vi "log in.vi"(0 "路径":path, 5 "UserGroups in":enum16{"Operator", "Engineer", "Admin"}(ring), 11 "error in (no error)":errorcluster caption="错误输入（无错误）") -> (4 "State":T1, 6 "Giveup?":bool, 8 "UserGroups":enum16{"Operator", "Engineer", "Admin"}(ring), 10 "User":string, 15 "error out":errorcluster caption="错误输出")   [LabVIEW 2017]
uses:
  Regedit.ctl
panel:
  in  "Exit":bool
  in  "Account":bool
  in  "Regist":bool
  in  "Login":bool
  in  "登录":T2
  # "Login"
  # "Tips\n1. Register new users for the user group (the administrator account cannot be registered)\n2. Select the user group;\n3. Enter the user name and password\n4, login"
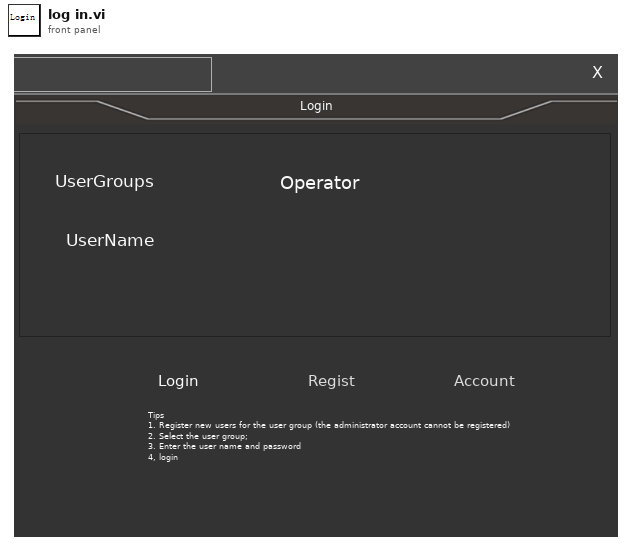
[diagram p1: front panel]
types:
  T1 = typedef "Regedit.ctl" = enum16{"Initialize", "Idle", "Judge", "Save", "Regedit", "Account", "Delete", "Sure?", "Stop"}
  T2 = cluster{"UserGroups":enum16{"Operator", "Engineer", "Admin"}, "UserName":string, "PassWord":string}
  T3 = enum8{"Enabled", "Disabled", "Disabled and Grayed Out"}
  T4 = enum16{"Operator", "Technician", "Engineer", "Developer"}
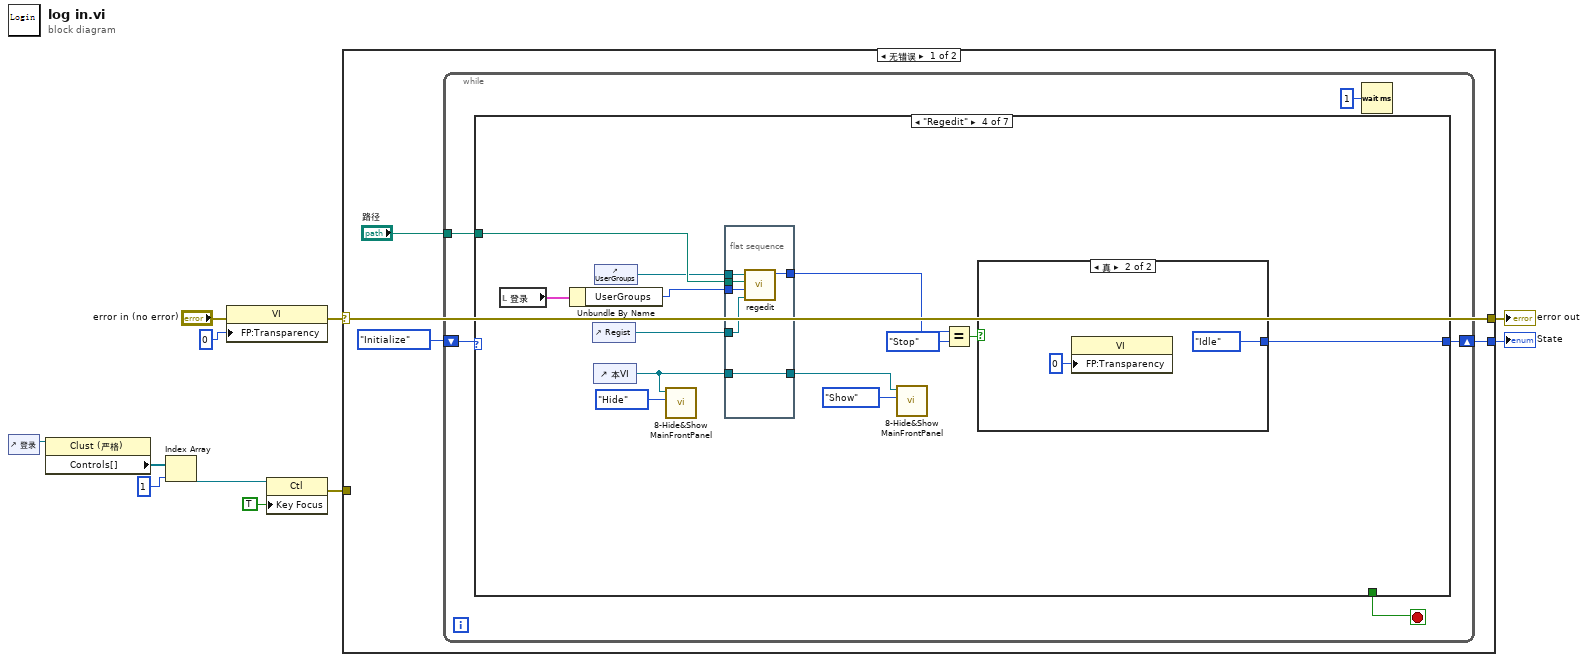
[diagram p0: block diagram]
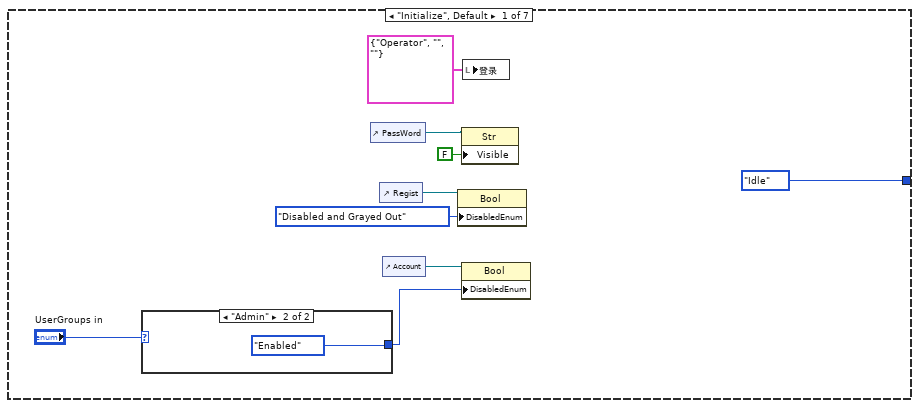
[diagram p2: hidden frame]
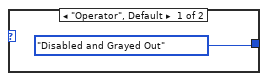
[diagram p3: hidden frame]
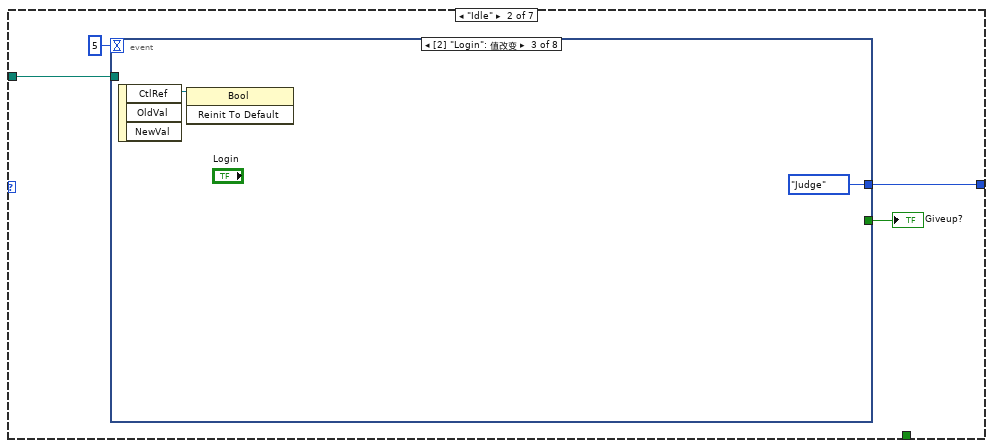
[diagram p4: hidden frame]
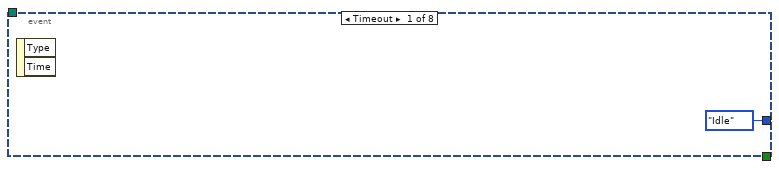
[diagram p5: hidden frame]
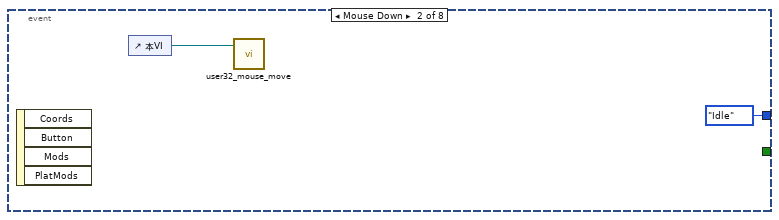
[diagram p6: hidden frame]
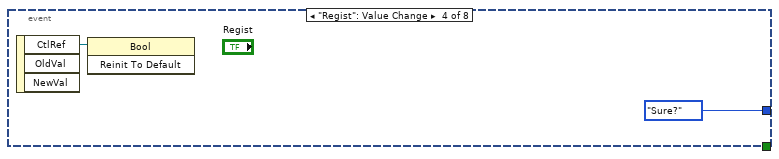
[diagram p7: hidden frame]
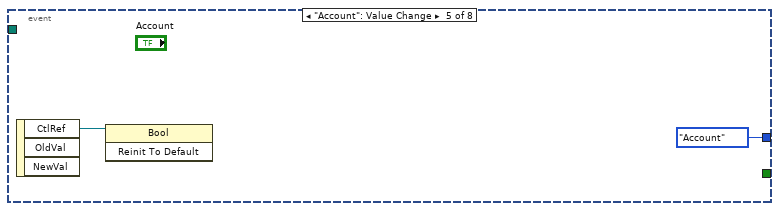
[diagram p8: hidden frame]
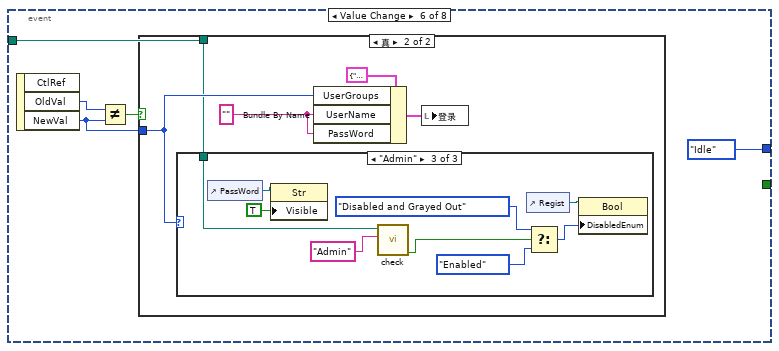
[diagram p9: hidden frame]
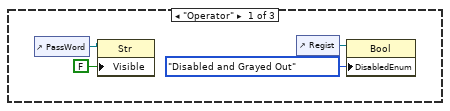
[diagram p11: hidden frame]
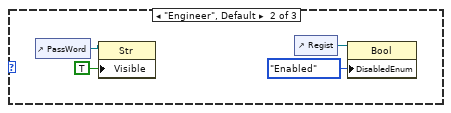
[diagram p12: hidden frame]
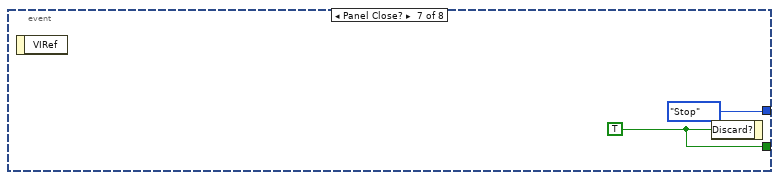
[diagram p13: hidden frame]
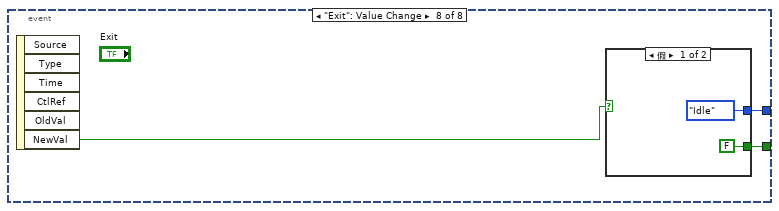
[diagram p14: hidden frame]
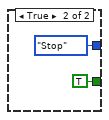
[diagram p15: hidden frame]
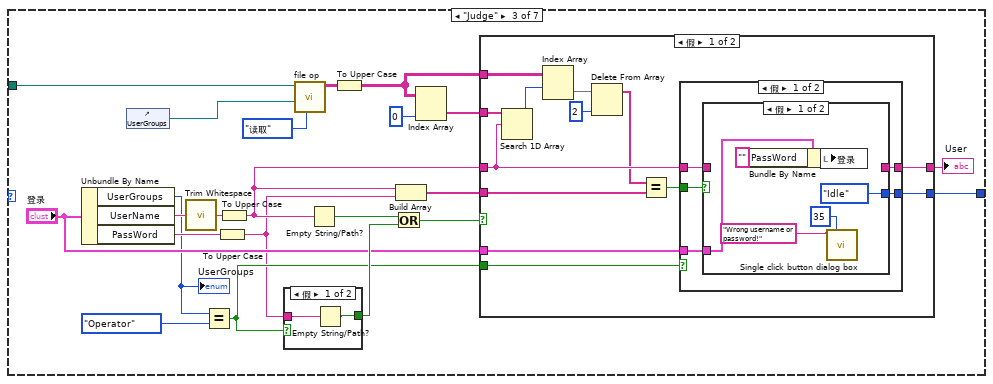
[diagram p16: hidden frame]
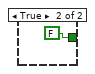
[diagram p17: hidden frame]
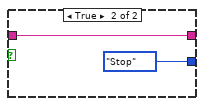
[diagram p18: hidden frame]
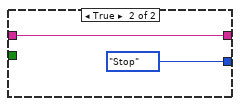
[diagram p19: hidden frame]
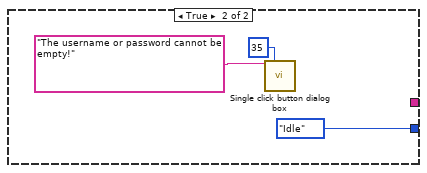
[diagram p20: hidden frame]
diagram:
  n1 = control-ref of="登录"() -> (w6:refnum<vi>)
  n2 = property class="Clust (严格)"(reference=w6) -> ("Controls[]"=w5:refnum<vi>[])  [unwired: 1 in, 2 out]
  n3 = Index Array(array=w5, index=1 ("索引")) -> (element=w3:refnum<vi>)
  n4 = property class="VI"(error in="error in (no error)", "FP:Transparency"=u8 0 ("前面板窗口:透明度")) -> (error out=w8:errorcluster)  [unwired: 1 in, 1 out]
  n5 = property class="Ctl"(reference=w3, "Key Focus"=TRUE ("键选中")) -> (error out=w1:errorcluster)  [unwired: 1 in, 1 out]
  n6 = case shown="无错误" w8 {
    selector: w8 -> [w14 w186]
    tunnel: [w14 w186] -> w11
    tunnel: [w13 _] -> w10
    tunnel: w1 -> [_ _]
    frame No Error {
      n7 = while {
        shift-right: [w19] -> w13
        shift-left: Regedit."Initialize" -> [w20]
        tunnel: "路径" -> [w17]
        stop <- w16 stop-if-true
        n8 = case shown="\"Regedit\"" w20 {
          tunnel: [Regedit."Idle" w34 w99 w146 Regedit."Idle" w168 Regedit."Stop"] -> w19
          tunnel: w17 -> [_ w32 w90 w145 w163 w169 _]
          tunnel: [_ _ _ _ _ _ TRUE] -> w16
          frame "Initialize", Default {
            n9 = case shown="\"Admin\"" "UserGroups in" {
              tunnel: [T3."Disabled and Grayed Out" ("禁用") T3."Enabled" ("禁用")] -> w22
              frame "Operator", Default {
              }
              frame "Admin" {
              }
            }
            n10 = control-ref of="PassWord"() -> (w28:refnum<vi>)
            n11 = control-ref of="Regist"() -> (w25:refnum<vi>)
            n12 = control-ref of="Account"() -> (w24:refnum<vi>)
            n13 = property class="Bool"(reference=w25, "DisabledEnum"=T3."Disabled and Grayed Out" ("禁用")) -> ()  [unwired: 1 in, 2 out]
            n14 = property class="Str"(reference=w28, "Visible"=FALSE ("可见")) -> ()  [unwired: 1 in, 2 out]
            n15 = property class="Bool"(reference=w24, "DisabledEnum"=w22) -> ()  [unwired: 1 in, 2 out]
            n16 = local write "登录"(T2 {"UserGroups"=enum."Operator", "UserName"="", "PassWord"=""} ("登录")) -> ()
          }
          frame "Idle" {
            n17 = event shown="[2] \"Login\": 值改变" {
              selector: _ -> [_ _ _ _ _ _ _ _]
              dyn-events: _ -> [_ _ _ _ _ _ _ _]
              timeout: 5 -> [_ _ _ _ _ _ _ _]
              tunnel: [Regedit."Idle" Regedit."Idle" Regedit."Judge" Regedit."Sure?" Regedit."Account" Regedit."Idle" Regedit."Stop" w76] -> w34
              tunnel: [_ _ _ _ _ _ w72 w75] -> w33
              tunnel: w32 -> [_ _ _ _ _ w45 _ _]
              event Timeout {
                n18 = event-data() -> ()  [unwired: 1 in, 2 out]
              }
              event Mouse Down {
                n19 = event-data() -> ()  [unwired: 1 in, 4 out]
                n20 = control-ref of="本VI"() -> (w37:refnum<vi>)
                n21 = call "user32_mouse_move.vi"("VI输入"=w37) -> ()  [unwired: 11 in]
              }
              event "Login": Value Change {
                n22 = event-data() -> ("CtlRef"=w40:refnum<vi>)  [unwired: 1 in, 2 out]
                n23 = invoke class="Bool" method="Reinit To Default"(reference=w40) -> ()  [unwired: 2 in, 3 out]
              }
              event "Regist": Value Change {
                n24 = event-data() -> ("CtlRef"=w42:refnum<vi>)  [unwired: 1 in, 2 out]
                n25 = invoke class="Bool" method="Reinit To Default"(reference=w42) -> ()  [unwired: 2 in, 3 out]
              }
              event "Account": Value Change {
                n26 = event-data() -> ("CtlRef"=w44:refnum<vi>)  [unwired: 1 in, 2 out]
                n27 = invoke class="Bool" method="Reinit To Default"(reference=w44) -> ()  [unwired: 2 in, 3 out]
              }
              event "登录.UserGroups": Value Change {
                n28 = event-data() -> ("OldVal"=w49:enum16{"Operator", "Engineer", "Admin"}, "NewVal"=w46:enum16{"Operator", "Engineer", "Admin"})  [unwired: 1 in, 1 out]
                n29 = Not Equal?(x=w49, y=w46) -> (x != y?=w47:bool)
                n30 = case shown="真" w47 {
                  tunnel: w46 -> [_ w51]
                  tunnel: w45 -> [_ w50]
                  frame False {
                  }
                  frame True {
                    w54 = "" ("用户名")
                    n31 = case shown="\"Admin\"" w51 {
                      tunnel: w50 -> [_ _ w67]
                      frame "Operator" {
                        n32 = control-ref of="PassWord"() -> (w58:refnum<vi>)
                        n33 = property class="Str"(reference=w58, "Visible"=FALSE ("可见")) -> ()  [unwired: 1 in, 2 out]
                        n34 = control-ref of="Regist"() -> (w55:refnum<vi>)
                        n35 = property class="Bool"(reference=w55, "DisabledEnum"=T3."Disabled and Grayed Out" ("禁用")) -> ()  [unwired: 1 in, 2 out]
                      }
                      frame "Engineer", Default {
                        n36 = control-ref of="PassWord"() -> (w62:refnum<vi>)
                        n37 = property class="Str"(reference=w62, "Visible"=TRUE ("可见")) -> ()  [unwired: 1 in, 2 out]
                        n38 = control-ref of="Regist"() -> (w59:refnum<vi>)
                        n39 = property class="Bool"(reference=w59, "DisabledEnum"=T3."Enabled" ("禁用")) -> ()  [unwired: 1 in, 2 out]
                      }
                      frame "Admin" {
                        n40 = control-ref of="PassWord"() -> (w71:refnum<vi>)
                        n41 = property class="Str"(reference=w71, "Visible"=TRUE ("可见")) -> ()  [unwired: 1 in, 2 out]
                        n42 = call "check.vi"("section"="Admin", "路径"=w67) -> ("存在？"=w66:bool)  [unwired: 9 in]
                        n43 = control-ref of="Regist"() -> (w69:refnum<vi>)
                        n44 = Select(t=T3."Disabled and Grayed Out" ("禁用"), s=w66, f=T3."Enabled" ("禁用")) -> (s? t:f=w65:T3)
                        n45 = property class="Bool"(reference=w69, "DisabledEnum"=w65) -> ()  [unwired: 1 in, 2 out]
                      }
                    }
                    n46 = Bundle By Name(cluster=T2 {"UserGroups"=enum."Operator", "UserName"="", "PassWord"=""} ("登录"), "UserGroups"=w51, "UserName"=w54, "PassWord"=w54) -> (w52:T2)
                    n47 = local write "登录"(w52) -> ()
                  }
                }
              }
              event Panel Close? {
                w72 = TRUE ("放弃？")
                n48 = event-data() -> ()  [unwired: 1 in, 1 out]
                n49 = event-data("Discard?"=w72) -> ()  [unwired: 1 in, 1 out]
              }
              event "Exit": Value Change {
                n50 = event-data() -> ("NewVal"=w74:bool)  [unwired: 1 in, 5 out]
                n51 = case shown="假" w74 {
                  tunnel: [Regedit."Idle" Regedit."Stop"] -> w76
                  tunnel: [FALSE ("放弃？") TRUE ("放弃？")] -> w75
                  frame False {
                  }
                  frame True {
                  }
                }
              }
            }
            "Giveup?" <- w33
          }
          frame "Judge" {
            n52 = Unbundle By Name("登录") -> ("UserGroups"=w87:enum16{"Operator", "Engineer", "Admin"}, "UserName"=w95:string, "PassWord"=w94:string)
            "UserGroups" <- w87
            n53 = control-ref of="UserGroups"() -> (w88:refnum<vi>)
            n54 = call <vilib>:"Trim Whitespace.vi"("string"=w95) -> ("trimmed string"=w81:string)  [unwired: 1 in]
            n55 = Equal?(x=w87, y=enum16{"Operator", "Engineer", "Admin"}."Operator") -> (x = y?=w85:bool)
            n56 = To Upper Case(1:w94) -> (0:w82:string)
            n57 = To Upper Case(1:w81) -> (0:w83:string)
            n58 = case shown="假" w85 {
              tunnel: [w104 FALSE] -> w101
              tunnel: w82 -> [w103 _]
              frame False {
                n59 = Empty String/Path?(string/path=w103) -> (empty?=w104:bool)
              }
              frame True {
              }
            }
            n60 = call "file op.vi"("操作"=enum16{"读取", "写入"}."读取", "UserGroups 2"=w88, "路径"=w90) -> ("添加的数组"=w96:string[][])  [unwired: 7 in, 1 out]
            n61 = Empty String/Path?(string/path=w83) -> (empty?=w102:bool)
            n62 = To Upper Case(1:w96) -> (0:w84:string[][])
            n63 = Or(x=w102, y=w101) -> (x .or. y?=w100:bool)
            n64 = Build Array(w83, w82) -> (w93:string[])
            n65 = Index Array(array=w84, index (col)=0 ("禁用的索引 (列)")) -> (element=w97:string[])  [unwired: 1 in]
            n66 = case shown="假" w100 {
              tunnel: [w112 Regedit."Idle"] -> w99
              tunnel: w97 -> [w118 _]
              tunnel: w83 -> [w111 _]
              tunnel: w84 -> [w117 _]
              tunnel: w93 -> [w106 _]
              tunnel: [w110 _] -> w92
              tunnel: "登录" -> [w109 _]
              tunnel: w85 -> [w108 _]
              frame False {
                n67 = Search 1D Array(1D array=w118, element=w111) -> (index of element=w116:i32)  [unwired: 1 in]
                n68 = Index Array(array=w117, index (row)=w116) -> (element=w115:string[])  [unwired: 1 in]
                n69 = Delete From Array(array=w115, index=2 ("索引")) -> (array with subset deleted=w107:string[])  [unwired: 1 in, 1 out]
                n70 = Equal?(x=w107, y=w106) -> (x = y?=w113:bool)
                n71 = case shown="假" w108 {
                  tunnel: w113 -> [w123 _]
                  tunnel: [w122 Regedit."Stop"] -> w112
                  tunnel: w111 -> [w121 w133]
                  tunnel: [w120 w133] -> w110
                  tunnel: w109 -> [w119 _]
                  frame False {
                    n72 = case shown="假" w123 {
                      tunnel: [Regedit."Idle" Regedit."Stop"] -> w122
                      tunnel: w121 -> [_ w130]
                      tunnel: [_ w130] -> w120
                      tunnel: w119 -> [w128 _]
                      frame False {
                        n73 = Bundle By Name(cluster=w128, "PassWord"="" ("密码")) -> (w126:T2)
                        n74 = local write "登录"(w126) -> ()
                        n75 = call "Single click button dialog box.vi"("Out"="Wrong username or password!" ("消息"), "size"=u32 35) -> ()  [unwired: 12 in, 2 out]
                      }
                      frame True {
                      }
                    }
                  }
                  frame True {
                  }
                }
              }
              frame True {
                n76 = call "Single click button dialog box.vi"("Out"="The username or password cannot be empty!" ("消息"), "size"=u32 35) -> ()  [unwired: 12 in, 2 out]
              }
            }
            "User" <- w92
          }
          frame "Regedit" {
            n77 = local read "登录"() -> (w143:T2)
            n78 = Unbundle By Name(w143) -> ("UserGroups"=w142:enum16{"Operator", "Engineer", "Admin"})
            n79 = control-ref of="Regist"() -> (w137:refnum<vi>)
            n80 = control-ref of="本VI"() -> (w138:refnum<vi>)
            n81 = control-ref of="UserGroups"() -> (w144:refnum<vi>)
            n82 = call "8-Hide&Show MainFrontPanel.vi"("Hide&Show"=enum16{"Hide", "Show"}."Hide", "This VI"=w138) -> ()  [unwired: 9 in, 1 out]
            n83 = flat-sequence {
              tunnel: [w155] -> w149
              tunnel: w145 -> [w154]
              tunnel: w144 -> [w153]
              tunnel: w142 -> [w152]
              tunnel: [w151] -> w139
              tunnel: w138 -> [w151]
              tunnel: w137 -> [w150]
              frame #0 {
                n84 = call "regedit.vi"("Regist"=w150, "UserGroups"=w152, "路径"=w154, "UserGroups 2"=w153) -> ("State"=w155:T1)  [unwired: 7 in]
              }
            }
            n85 = call "8-Hide&Show MainFrontPanel.vi"("Hide&Show"=enum16{"Hide", "Show"}."Show", "This VI"=w139) -> ()  [unwired: 9 in, 1 out]
            n86 = Equal?(x=w149, y=Regedit."Stop") -> (x = y?=w147:bool)
            n87 = case shown="真" w147 {
              tunnel: [Regedit."Regedit" Regedit."Idle"] -> w146
              frame False {
              }
              frame True {
                n88 = property class="VI"("FP:Transparency"=u8 0 ("前面板窗口:透明度")) -> ()  [unwired: 2 in, 2 out]
              }
            }
          }
          frame "Account" {
            n89 = control-ref of="本VI"() -> (w160:refnum<vi>)
            n90 = call "8-Hide&Show MainFrontPanel.vi"("Hide&Show"=enum16{"Hide", "Show"}."Hide", "This VI"=w160) -> ()  [unwired: 9 in, 1 out]
            n91 = flat-sequence {
              tunnel: w163 -> [w166]
              tunnel: w160 -> [w165]
              tunnel: [w165] -> w159
              frame #0 {
                n92 = call "Account.vi"("路径"=w166) -> ()  [unwired: 12 in, 3 out]
              }
            }
            n93 = call "8-Hide&Show MainFrontPanel.vi"("Hide&Show"=enum16{"Hide", "Show"}."Show", "This VI"=w159) -> ()  [unwired: 9 in, 1 out]
          }
          frame "Sure?" {
            n94 = local read "登录"() -> (w171:T2)
            n95 = Unbundle By Name(w171) -> ("UserGroups"=w170:enum16{"Operator", "Engineer", "Admin"})
            n96 = Equal?(x=w170, y=T4."Developer" ("UserGroups")) -> (x = y?=w172:bool)
            n97 = case shown="真" w172 {
              tunnel: [Regedit."Regedit" w177] -> w168
              tunnel: w170 -> [_ _]
              tunnel: w169 -> [_ w176]
              frame False {
                n98 = control-ref of="本VI"() -> (w173:refnum<vi>)
                n99 = property class="VI"(reference=w173, "FP:Transparency"=u8 100 ("前面板窗口:透明度")) -> ()  [unwired: 1 in, 2 out]
              }
              frame True {
                n100 = call "check.vi"("section"="Admin", "路径"=w176) -> ("存在？"=w178:bool)  [unwired: 9 in]
                n101 = case shown="真" w178 {
                  tunnel: [Regedit."Regedit" Regedit."Idle"] -> w177
                  frame False {
                  }
                  frame True {
                    n102 = call "Single click button dialog box.vi"("Out"="The Admin account already exists and cannot be registered!" ("消息"), "size"=u32 25) -> ()  [unwired: 12 in, 2 out]
                  }
                }
              }
            }
          }
          frame "Stop" {
          }
        }
        n103 = Wait (ms)(milliseconds to wait=u32 1) -> ()  [unwired: 1 out]
      }
    }
    frame Error {
    }
  }
  "error out" <- w11
  "State" <- w10
